vi "CC Post-Build Action.vi"(5 "Files Generated by Build":path[](array[path]), 6 "Top Level/Always Included VIs":path[](array[path]), 7 "Destination Path":path, 8 "error in (no error)":errorcluster, 9 "Target Name":string, 10 "Build Specification Name":string, 11 "Project Path":path) -> (0 "error out":errorcluster)   [LabVIEW 2021]
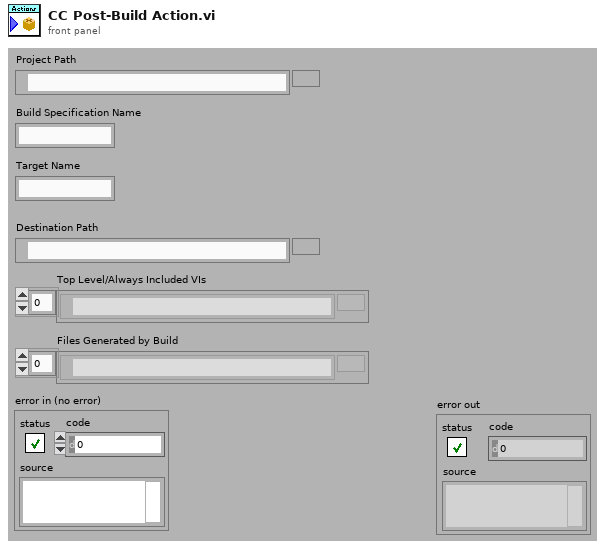
[diagram p1: front panel]
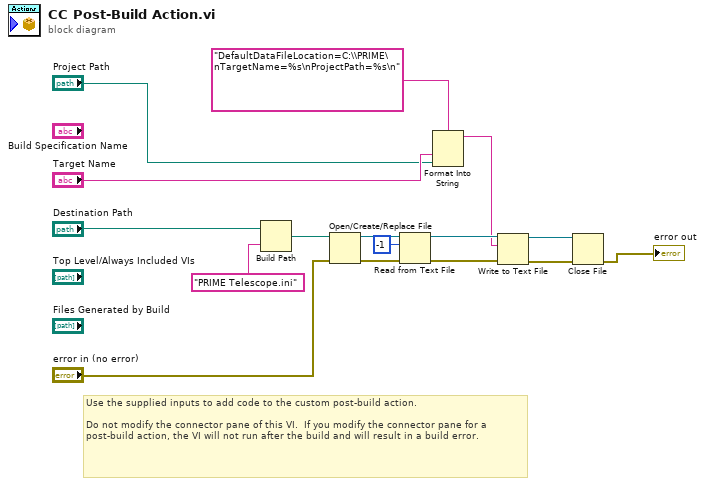
[diagram p0: block diagram]
diagram:
  # "Use the supplied inputs to add code to the custom post-build action.\n\nDo not modify the connector pane of this VI.  If you modify the connector pane for a post-build action, the VI will not run after the build and will result in a build error."
  n1 = Build Path(base path="Destination Path", name or relative path="PRIME Telescope.ini") -> (appended path=w14:path)
  n2 = Open/Create/Replace File(file path (use dialog)=w14, error in="error in (no error)") -> (refnum out=w8:refnum<file>, error out=w9:errorcluster)  [unwired: 4 in, 1 out]
  n3 = Read from Text File(file (use dialog)=w8, count=-1, error in=w9) -> (refnum out=w6:refnum<file>, error out=w5:errorcluster)  [unwired: 1 in, 2 out]
  n4 = Format Into String(format string="DefaultDataFileLocation=C:\\PRIME\nTargetName=%s\nProjectPath=%s\n" ("key"), "Target Name", "Project Path") -> (resulting string=w4:string)  [unwired: 2 in, 1 out]
  n5 = Write to Text File(file (use dialog)=w6, text=w4, error in=w5) -> (refnum out=w12:refnum<file>, error out=w13:errorcluster)  [unwired: 1 in, 1 out]
  n6 = Close File(refnum=w12, error in=w13) -> (error out=→"error out":errorcluster)  [unwired: 1 out]
